vi "picoGetValues.vi"(4 "Down-Sample Mode":i32, 6 "Down Sample Ratio":u32, 7 "nCaptures":u16, 8 "error in (no error)":errorcluster, 9 "postTriggerSamples":u32, 11 "Handle In":i16) -> (0 "error out":errorcluster, 2 "buffer":i16[][](array[numeric]), 3 "handle":i16)   [LabVIEW 2011]
uses:
  PS2000a.dll
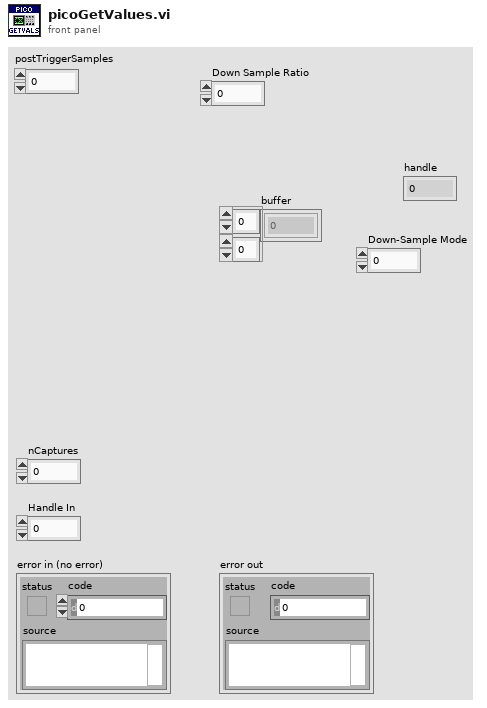
[diagram p1: front panel]
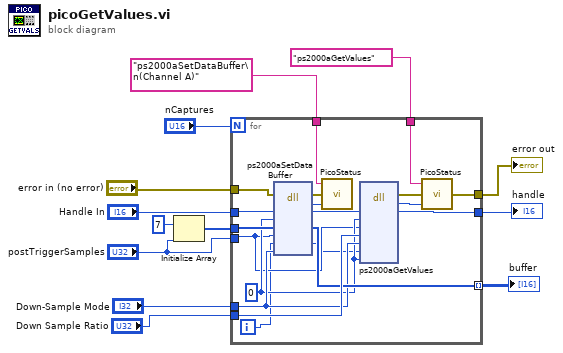
[diagram p0: block diagram]
diagram:
  n1 = Initialize Array(u16 7 ("element"), "postTriggerSamples") -> (w11:u16[])
  n2 = for {
    N: "nCaptures" -> [_]
    tunnel: "error in (no error)" -> [w15]
    tunnel: "Handle In" -> [w18]
    tunnel: "postTriggerSamples" -> [w17]
    tunnel: [w32] -> w9
    tunnel: [w27] -> w10
    tunnel: w11 -> [w20]
    tunnel: [w24] -> w12 mode=indexing
    tunnel: "Down-Sample Mode" -> [w21]
    tunnel: "Down Sample Ratio" -> [w31]
    tunnel: "ps2000aSetDataBuffer\n(Channel A)" ("source") -> [w30]
    tunnel: "ps2000aGetValues" ("source") -> [w26]
    i -> [w16]
    w19 = 0 ("channel")
    n3 = dll-call lib="ps2000a.dll" fn="ps2000aSetDataBuffer" ("ps3000.dll:_ps3000_open_unit@0")(error in=w15, "handle"=w18, "channel"=w19, "buffer"=w20, "bufferLth"=w17, "waveform"=w16, "downSampleRatioMode"=w21) -> (error out=w25:errorcluster, "PICO_STATUS"=w22:i32, "handle"=w23:i16, "buffer"=w24:i16[], "waveform"=w14:u32)  [unwired: 5 in, 1 out]
    n4 = call "PicoStatus.vi"("PICO STATUS"=w22, "error in"=w25, "source"=w30) -> ()  [unwired: 1 out]
    n5 = dll-call lib="ps2000a.dll" fn="ps2000aGetValues" ("ps3000.dll:_ps3000_open_unit@0")("handle"=w23, "startIndex"=w19, "noOfSamples"=w17, "downSampleRatio"=w31, "downSampleRatioMode"=w21, "segmentIndex"=w14, "overflow"=w19) -> (error out=w28:errorcluster, "PICO_STATUS"=w29:i32, "handle"=w32:i16)  [unwired: 9 in, 1 out]
    n6 = call "PicoStatus.vi"("PICO STATUS"=w29, "error in"=w28, "source"=w26) -> ("error out"=w27:errorcluster)
  }
  "buffer" <- w12
  "error out" <- w10
  "handle" <- w9
